vi "read_time_const.vi"(1 "VISA session (for class)":refnum<visa-resource-name>) -> (0 "time_const":string)   [LabVIEW 2015]
doc: "This VI reads the time constant of the Lock-In."
panel:
  out "XTC":i32
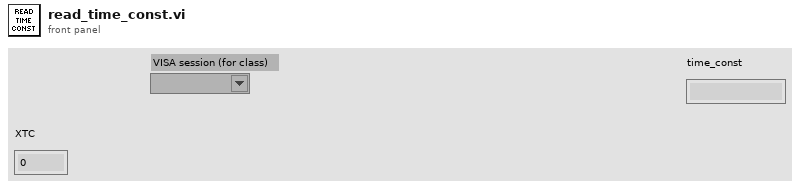
[diagram p1: front panel]
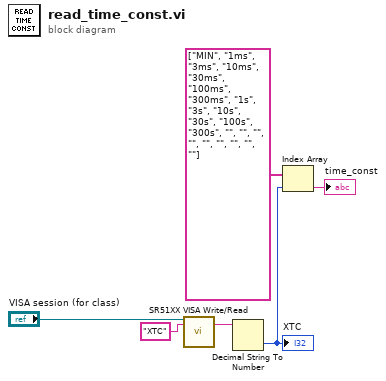
[diagram p0: block diagram]
diagram:
  n1 = call "SR51XX VISA Write/Read"("VISA session (for class)"="VISA session (for class)", "Write Command String"="XTC") -> ("Response 1"=w5:string)  [unwired: 6 in, 11 out]
  n2 = Decimal String To Number(string=w5) -> (number=w3:i32)  [unwired: 2 in, 1 out]
  "XTC" <- w3
  n3 = Index Array(array=string[] ["MIN", "1ms", "3ms", "10ms", "30ms", "100ms", "300ms", "1s", "3s", "10s", "30s", "100s", "300s", "", "", "", "", "", "", "", "", ""], index=w3) -> (element=→"time_const":string)
